vi "3DVisPrep.vi"() -> ()   [LabVIEW 2022 SP3]
uses:
  <vilib>/Utility/file.llb/Read From Spreadsheet File (DBL).vi
  <vilib>/Utility/file.llb/Write To Spreadsheet File (DBL).vi
panel:
  in  "reduce pts by factor of":u8=1
  out "Array":u8[][][](array[numeric])
  in  "Image Size":cluster{"Width":u32, "Height":u32}
  in  "name of saved file":string="test"
  out "Pict Images (if any)":picture[](array[picture])
  out "BMP Dimensions":T1(array[cluster])
  in  "Choose Directory of Files":path=path "C:/WINDOWS/DESKTOP/rri.eye"
  in  "How to save data":u16(ring) items=["X Y Z value + param in spreadsheet", "Save spreadsheet planes as 8 bit byte planes", "Save spreadsheet planes as single byte file", "save spreadsheet planes as 8 bit bitmaps", "Save RGB BMP planes as one 8 bit byte file (Ernie's BMP)", "Save RGB BMP planes as 8 bit BMP files (Ernie's BMP)", "Save RGB BMP planes as one 8 bit byte file specify pixels in X and Y (Fred's BMP)", "Convert eye file to 8 bit unsigned byte file. Reduce points if desired"]
  out "Dimensions (Z,Y,X)":i32[](array[numeric])
  in  "Number of files":i32
  in  "Root name of file":string="plane"
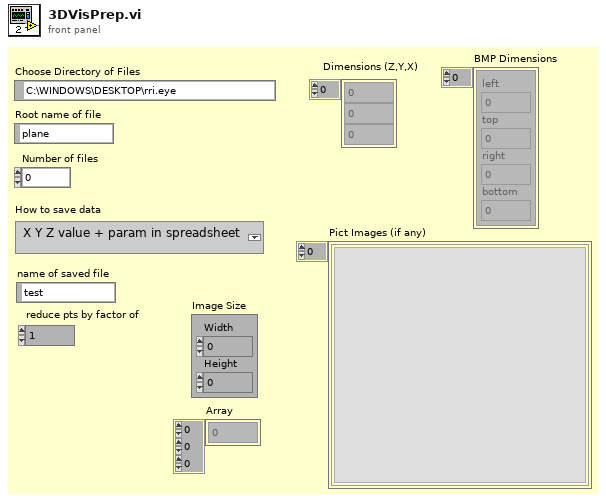
[diagram p1: front panel]
types:
  T1 = cluster{"left":i16, "top":i16, "right":i16, "bottom":i16}[]
  T2 = cluster{"left":i16, "top":i16, "right":i16, "bottom":i16}
  T3 = enum32{"existing file", "new file", "new or existing file", "existing dir", "new dir", "new or existing dir", "existing file (use LLBs)", "new file (use LLBs)", "new or existing file (use LLBs)", "new or existing file or directory (use LLBs)"}
  T4 = enum16{"open", "open or create", "create or replace", "create"}
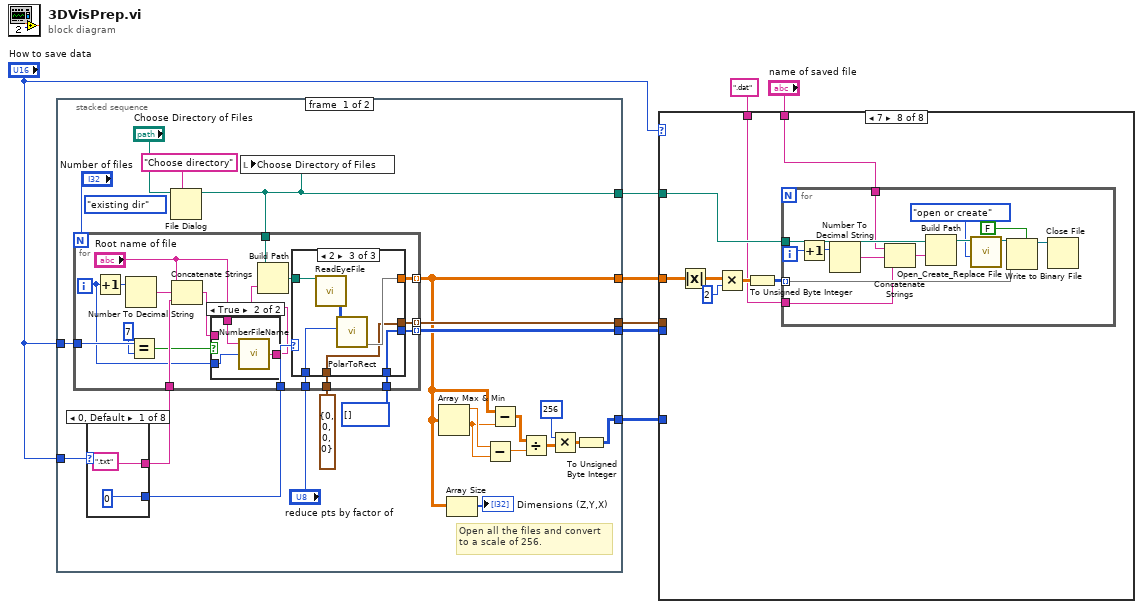
[diagram p0: block diagram]
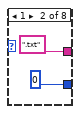
[diagram p2: hidden frame]
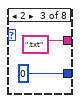
[diagram p3: hidden frame]
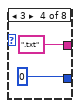
[diagram p4: hidden frame]
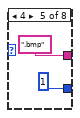
[diagram p5: hidden frame]
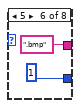
[diagram p6: hidden frame]
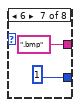
[diagram p7: hidden frame]
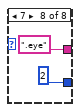
[diagram p8: hidden frame]
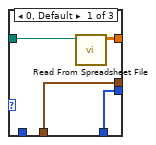
[diagram p10: hidden frame]
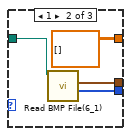
[diagram p11: hidden frame]
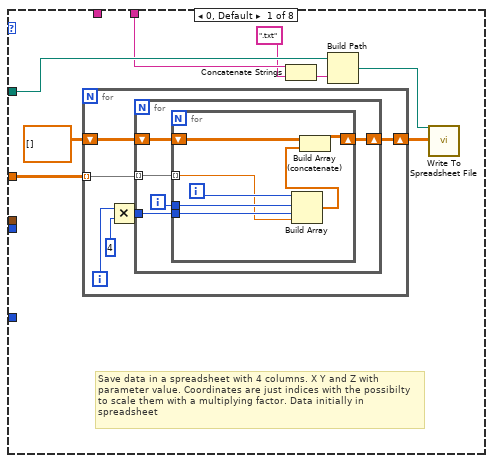
[diagram p13: hidden frame]
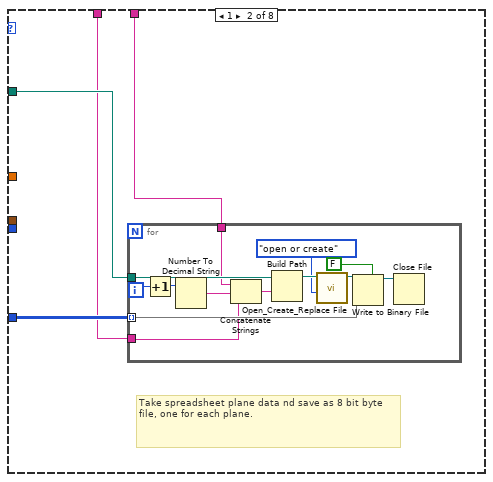
[diagram p14: hidden frame]
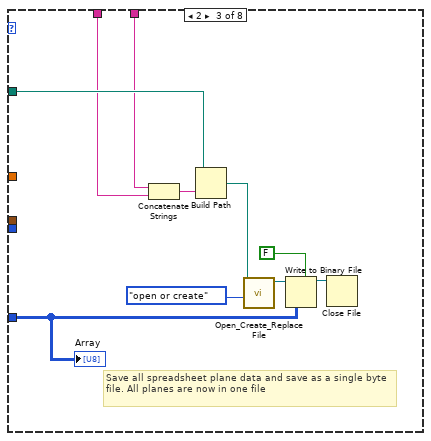
[diagram p15: hidden frame]
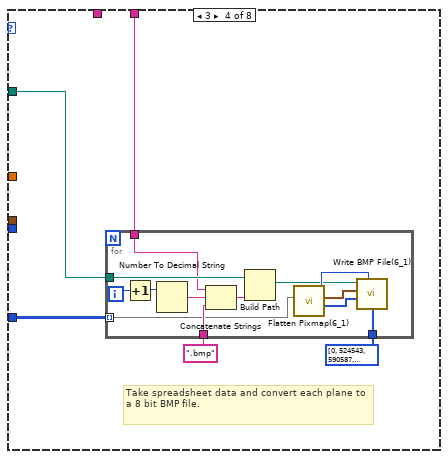
[diagram p16: hidden frame]
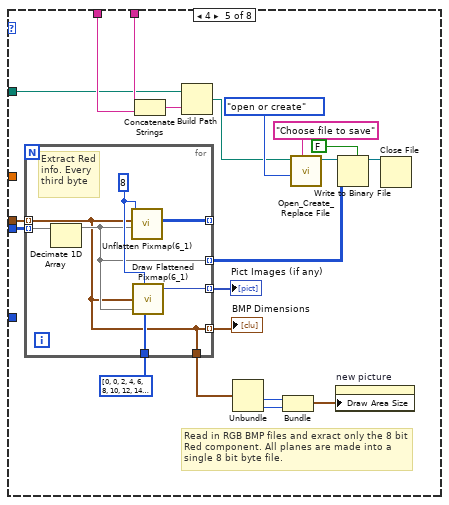
[diagram p17: hidden frame]
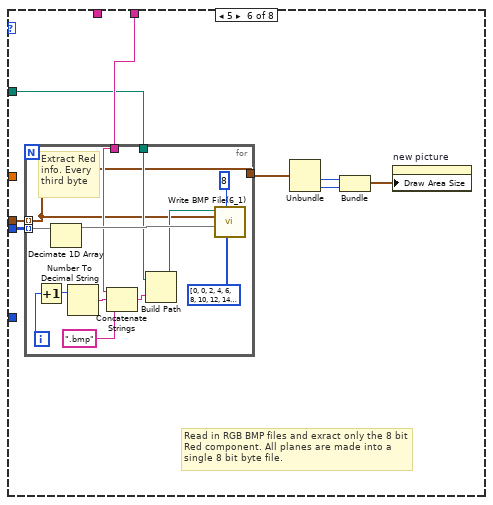
[diagram p18: hidden frame]
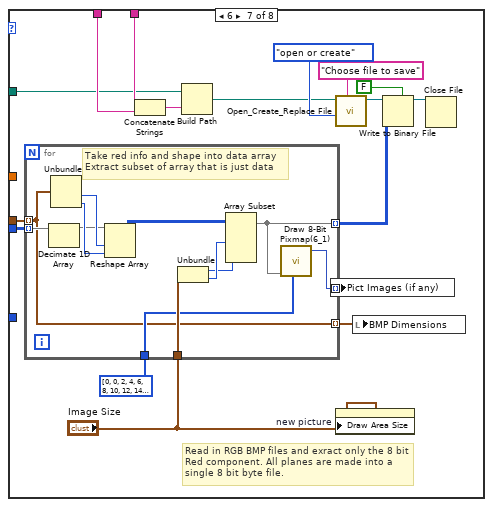
[diagram p19: hidden frame]
diagram:
  n1 = stacked-sequence {
    tunnel: [w27 _] -> w8
    tunnel: [w21 _] -> w7
    tunnel: [w17 _] -> w6
    tunnel: [w26 _] -> w5
    tunnel: [w25 _] -> w4
    tunnel: "How to save data" -> [w15 _]
    tunnel: "How to save data" -> [w10 _]
    frame #0 {
      (unwired) T3."existing dir" ("select mode (2)")
      # "Open all the files and convert\nto a scale of 256."
      n2 = case shown="0, Default" w15 {
        tunnel: [".txt" ".txt" ".txt" ".txt" ".bmp" ".bmp" ".bmp" ".eye"] -> w14
        tunnel: [0 0 0 0 1 1 1 2] -> w13
        frame 0, Default {
        }
        frame 1 {
        }
        frame 2 {
        }
        frame 3 {
        }
        frame 4 {
        }
        frame 5 {
        }
        frame 6 {
        }
        frame 7 {
        }
      }
      n3 = File Dialog(7:"Choose directory" ("prompt"), 11:"Choose Directory of Files") -> (3:w27:path)  [unwired: 5 in, 3 out]
      n4 = for {
        N: "Number of files" -> [_]
        tunnel: w27 -> [w65]
        tunnel: [w63] -> w21 mode=indexing
        tunnel: [w62] -> w26 mode=indexing
        tunnel: [w61] -> w25 mode=indexing
        tunnel: w14 -> [w60]
        tunnel: w13 -> [w59]
        tunnel: u8[] [] ("Array Constant") -> [w58]
        tunnel: T2 {"left"=0, "top"=0, "right"=0, "bottom"=0} ("rect") -> [w57]
        tunnel: w10 -> [w55]
        tunnel: "reduce pts by factor of" -> [w49]
        i -> [w50]
        n5 = Increment(x=w50) -> (x+1=w51:i32)
        n6 = Number To Decimal String(number=w51) -> (decimal integer string=w66:string)  [unwired: 1 in]
        n7 = Equal?(x=w55, y=7) -> (x = y?=w56:bool)
        n8 = Concatenate Strings("Root name of file", w66, w60) -> (w53:string)
        n9 = case shown="True" w56 {
          tunnel: [w67 w70] -> w48
          tunnel: w53 -> [w67 _]
          tunnel: "Root name of file" -> [_ w69]
          tunnel: w50 -> [_ w68]
          frame False {
          }
          frame True {
            n10 = call "NumberFileName.vi"("File number"=w68, "file name"=w69) -> ("Numbered File"=w70:string)  [unwired: 1 in]
          }
        }
        n11 = Build Path(base path=w65, name or relative path=w48) -> (appended path=w64:path)
        n12 = case shown="2" w59 {
          tunnel: w64 -> [w74 w78 w84]
          tunnel: [w73 dbl[][] [] ("Array Constant") w82] -> w63
          tunnel: [w72 w77 w81] -> w62
          tunnel: [w71 w75 w80] -> w61
          tunnel: w58 -> [w72 _ w81]
          tunnel: w57 -> [w71 _ w80]
          tunnel: w49 -> [_ _ w79]
          frame 0, Default {
            n13 = call-poly <vilib>:"Read From Spreadsheet File.vi"("file path (dialog if empty)"=w74) -> ("all rows"=w73:dbl[][])  [unwired: 6 in, 4 out]
          }
          frame 1 {
            n14 = call <vilib>:"Read BMP File(6_1).vi"("path to BMP file"=w78) -> ("flattened image data"=w77:u8[], "rect"=w75:T2)  [unwired: 5 in, 4 out]
          }
          frame 2 {
            n15 = call "ReadEyeFile.vi"("new file path"=w84) -> ("2-D data array"=w83:i16[][])  [unwired: 10 in, 8 out]
            n16 = call "PolarToRect.vi"("c m/s"=w79, "array dims"=w83) -> (0:w82)  [unwired: 3 in, 6 out]
          }
        }
      }
      n17 = local write "Choose Directory of Files"(w27) -> ()
      n18 = Array Max & Min(array=w21) -> (max value=w24:dbl, min value=w23:dbl)  [unwired: 2 out]
      n19 = Array Size(array=w21) -> (size(s)=→"Dimensions (Z,Y,X)":i32[])
      n20 = Subtract(x=w24, y=w23) -> (x-y=w22:dbl)
      n21 = Subtract(x=w21, y=w23) -> (x-y=w20:dbl[][][])
      n22 = Divide(x=w20, y=w22) -> (x/y=w19:dbl[][][])
      n23 = Multiply(x=256, y=w19) -> (x*y=w16:dbl[][][])
      n24 = To Unsigned Byte Integer(number=w16) -> (unsigned 8bit integer=w17:u8[][][])
    }
    frame #1 {
    }
  }
  n25 = case shown="7" "How to save data" {
    tunnel: w8 -> [w89 w114 w133 w142 w162 w183 w210 w235]
    tunnel: w7 -> [w90 _ _ _ _ _ _ w240]
    tunnel: w6 -> [_ w113 w129 w139 _ _ _ _]
    tunnel: w5 -> [_ _ _ _ w175 w190 w220 _]
    tunnel: w4 -> [_ _ _ _ w174 w189 w219 _]
    tunnel: "name of saved file" -> [w87 w112 w132 w138 w164 w184 w212 w234]
    tunnel: ".dat" -> [_ w111 w131 _ w163 _ w211 w233]
    frame 0, Default {
      # "Save data in a spreadsheet with 4 columns. X Y and Z with parameter value. Coordinates are just indices with the possibilty\nto scale them with a multiplying factor. Data initially in spreadsheet"
      n26 = for {
        shift-right: [w98] -> w91
        shift-left: dbl[][] [] ("Array Constant") -> [w97]
        tunnel: w90 -> [w93] mode=indexing
        i -> [w95]
        n27 = Multiply(x=w95, y=4) -> (x*y=w94:i32)
        n28 = for {
          tunnel: w93 -> [w103] mode=indexing
          tunnel: w94 -> [w101]
          shift-right: [w100] -> w98
          shift-left: w97 -> [w99]
          i -> [w102]
          n29 = for {
            tunnel: w103 -> [w107] mode=indexing
            tunnel: w102 -> [w109]
            tunnel: w101 -> [w110]
            shift-right: [w105] -> w100
            shift-left: w99 -> [w106]
            i -> [w108]
            n30 = Build Array(w108, w109, w110, w107) -> (w104:dbl[])
            n31 = Build Array (concatenate)(w106, w104) -> (w105:dbl[][])
          }
        }
      }
      n32 = Concatenate Strings(w87, ".txt") -> (w86:string)
      n33 = Build Path(base path=w89, name or relative path=w86) -> (appended path=w88:path)
      n34 = call-poly <vilib>:"Write To Spreadsheet File.vi"("2D data"=w91, "file path (dialog if empty)"=w88) -> ()  [unwired: 6 in, 1 out]
    }
    frame 1 {
      # "Take spreadsheet plane data nd save as 8 bit byte file, one for each plane."
      n35 = for {
        tunnel: w113 -> [w121] mode=indexing
        tunnel: w114 -> [w120]
        tunnel: w112 -> [w119]
        tunnel: w111 -> [w117]
        i -> [w127]
        n36 = Increment(x=w127) -> (x+1=w126:i32)
        n37 = Number To Decimal String(number=w126) -> (decimal integer string=w118:string)  [unwired: 1 in]
        n38 = Concatenate Strings(w119, w118, w117) -> (w116:string)
        n39 = Build Path(base path=w120, name or relative path=w116) -> (appended path=w125:path)
        n40 = call <vilib>:"Open_Create_Replace File.vi"("function (open:0)"=T4."open or create", "file path"=w125) -> ("refnum"=w124:refnum<file>)  [unwired: 6 in, 3 out]
        n41 = Write to Binary File(file (use dialog)=w124, data=w121, 5:FALSE ("prepend array or string size? (T)")) -> (refnum out=w123:refnum<file>)  [unwired: 3 in, 2 out]
        n42 = Close File(refnum=w123) -> ()  [unwired: 1 in, 2 out]
      }
    }
    frame 2 {
      # "Save all spreadsheet plane data and save as a single byte file. All planes are now in one file"
      n43 = Concatenate Strings(w132, w131) -> (w134:string)
      n44 = Build Path(base path=w133, name or relative path=w134) -> (appended path=w130:path)
      n45 = call <vilib>:"Open_Create_Replace File.vi"("function (open:0)"=T4."open or create", "file path"=w130) -> ("refnum"=w136:refnum<file>)  [unwired: 6 in, 3 out]
      n46 = Write to Binary File(file (use dialog)=w136, data=w129, 5:FALSE ("prepend array or string size? (T)")) -> (refnum out=w137:refnum<file>)  [unwired: 3 in, 2 out]
      n47 = Close File(refnum=w137) -> ()  [unwired: 1 in, 2 out]
      "Array" <- w129
    }
    frame 3 {
      # "Take spreadsheet data and convert each plane to a 8 bit BMP file."
      n48 = for {
        tunnel: w139 -> [w147] mode=indexing
        tunnel: w142 -> [w153]
        tunnel: ".bmp" -> [w151]
        tunnel: u32[] [0, 524543, 590587, 591095, 657139, 657647, 723691, 724455, 790500, 791008, 857052, 923096, 923604, 989648, 990156, 1056200, 1056708, 1122752, 1123516, 1189560, 1255604, 1256113, 1322157, 1322665, 1388709, 1389217, 1455261, 1521305, 1521816, 1588120, 1588631, 1654678, 1655190, 1721237, 1721748, 1787796, 1853843, 1854354, 1920402, 1920913, 1987216, 1987728, 2053775, 2054286, 2120334, 2186381, 2186892, 2252940, 2253451, 2319498, 2320009, 2386313, 2386824, 2452871, 2518919, 2519430, 2585477, 2585989, 2652036, 2652547, 2718595, 2719106, 2785409, 2851457, 2851968, 2918015, 2918527, 2984574, 2985085, 3051133, 3051644, 3117691, 3183739, 3184250, 3250553, 3251065, 3317112, 3317623, 3383671, 3449718, 3450229, 3516277, 3516788, 3582835, 3583347, 3649650, 3650161, 3716209, 3782256, 3782767, 3848815, 3849326, 3915373, 3915885, 3981932, 3982443, 4048746, 4114794, 4115305, 4181352, 4181864, 4247911, 4248422, 4314470, 4314981, 4381028, 4447076, 4447843, 4513890, 4514402, 4580449, 4580960, 4647008, 4647519, 4713566, 4779614, 4780125, 4846172, 4846940, 4912987, 4913498, 4979546, 5045593, 5046104, 5111128, 5110615, 5175638, 5175126, 5240149, 5239636, 5304660, 5369683, 5369170, 5434450, 5433937, 5498960, 5498448, 5563471, 5562958, 5627982, 5693005, 5823564, 5888587, 6019147, 6084170, 6214729, 6279753, 6410312, 6475335, 6605895, 6670918, 6801477, 6866757, 6997316, 7062339, 7192899, 7257922, 7388481, 7453505, 7584064, 7649087, 7779647, 7844670, 7909693, 8040253, 8105276, 8235835, 8300859, 8431418, 8496441, 8627257, 8692280, 8822839, 8887863, 9018422, 9083445, 9214005, 9279028, 9409587, 9474611, 9605170, 9670193, 9800753, 9865776, 9996335, 10061359, 10126382, 10256941, 10321964, 10452780, 10517803, 10648362, 10713386, 10843945, 10908968, 11039528, 11104551, 11235110, 11300134, 11430693, 11495716, 11626276, 11691299, 11821858, 11886882, 12017441, 12082464, 12213024, 12278303, 12343326, 12473886, 12538909, 12669468, 12734492, 12865051, 12930074, 13060634, 13125657, 13256216, 13321240, 13451799, 13516822, 13647382, 13712405, 13842964, 13907988, 14038803, 14103826, 14234386, 14299409, 14429968, 14494992, 14560015, 14690574, 14755597, 14886157, 14951180, 15081739, 15146763, 15277322, 15342345, 15472905, 15537928, 15668487, 15733511, 15864326, 15929349, 16059909, 16124932, 16255491, 16320515, 16451074, 16516097, 16646657, 16711680, 16711680] -> [w144]
        tunnel: w138 -> [w143]
        i -> [w155]
        n49 = Increment(x=w155) -> (x+1=w154:i32)
        n50 = Number To Decimal String(number=w154) -> (decimal integer string=w152:string)  [unwired: 1 in]
        n51 = Concatenate Strings(w143, w152, w151) -> (w150:string)
        n52 = Build Path(base path=w153, name or relative path=w150) -> (appended path=w148:path)
        n53 = call <vilib>:"Flatten Pixmap(6_1).vi"("8-bit pixmap"=w147) -> ("flattened image data"=w145:u8[], "bounds"=w146:T2, "bit depth"=w149:u8)  [unwired: 8 in]
        n54 = call <vilib>:"Write BMP File(6_1).vi"("color table"=w144, "depth"=w149, "flattened image data"=w145, "rect"=w146, "path to BMP file"=w148) -> ()  [unwired: 5 in, 2 out]
      }
    }
    frame 4 {
      # "Read in RGB BMP files and exract only the 8 bit Red component. All planes are made into a single 8 bit byte file."
      n55 = for {
        tunnel: w175 -> [w181] mode=indexing
        tunnel: w174 -> [w176] mode=indexing
        tunnel: [w180] -> w167 mode=indexing
        tunnel: [w176] -> w173 mode=indexing
        tunnel: u32[] [0, 0, 2, 4, 6, 8, 10, 12, 14, 16, 18, 20, 22, 24, 26, 28, 30, 32, 34, 36, 38, 40, 42, 44, 46, 48, 50, 52, 54, 56, 58, 60, 62, 64, 66, 68, 70, 72, 74, 76, 78, 80, 82, 84, 86, 88, 90, 92, 94, 96, 98, 100, 102, 104, 106, 108, 110, 112, 114, 116, 118, 120, 122, 124, 126, 128, 130, 132, 134, 136, 138, 140, 142, 144, 146, 148, 150, 152, 154, 156, 158, 160, 162, 164, 166, 168, 170, 172, 174, 176, 178, 180, 182, 184, 186, 188, 190, 192, 194, 196, 198, 200, 202, 204, 206, 208, 210, 212, 214, 216, 218, 220, 222, 224, 226, 228, 230, 232, 234, 236, 238, 240, 242, 244, 246, 248, 250, 252, 255, 131839, 263423, 395007, 526591, 658175, 789759, 921343, 1052927, 1184511, 1316095, 1447679, 1579263, 1710847, 1842431, 1974015, 2105599, 2237183, 2368767, 2500351, 2631935, 2763519, 2895103, 3026687, 3158271, 3289855, 3421439, 3553023, 3684607, 3816191, 3947775, 4079359, 4210943, 4342527, 4474111, 4605695, 4737279, 4868863, 5000447, 5132031, 5263615, 5395199, 5526783, 5658367, 5789951, 5921535, 6053119, 6184703, 6316287, 6447871, 6579455, 6711039, 6842623, 6974207, 7105791, 7237375, 7368959, 7500543, 7632127, 7763711, 7895295, 8026879, 8158463, 8290047, 8421631, 8553215, 8684799, 8816383, 8947967, 9079551, 9211135, 9342719, 9474303, 9605887, 9737471, 9869055, 10000639, 10132223, 10263807, 10395391, 10526975, 10658559, 10790143, 10921727, 11053311, 11184895, 11316479, 11448063, 11579647, 11711231, 11842815, 11974399, 12105983, 12237567, 12369151, 12500735, 12632319, 12763903, 12895487, 13027071, 13158655, 13290239, 13421823, 13553407, 13684991, 13816575, 13948159, 14079743, 14211327, 14342911, 14474495, 14606079, 14737663, 14869247, 15000831, 15132415, 15263999, 15395583, 15527167, 15658751, 15790335, 15921919, 16053503, 16185087, 16316671, 16448255, 16579839, 16711680] ("Array 3") -> [w179]
        tunnel: [w178] -> _ mode=indexing
        tunnel: [w177] -> w166 mode=indexing
        tunnel: [w176] -> w158
        w182 = 8
        # "Extract Red\ninfo. Every \nthird byte"
        n56 = Decimate 1D Array(w181) -> (w180:u8[])  [unwired: 2 out]
        n57 = call <vilib>:"Unflatten Pixmap(6_1).vi"("flattened image data"=w180, "rect"=w176, "depth"=w182) -> ("8-bit pixmap"=w178:u8[][])  [unwired: 4 in, 4 out]
        n58 = call <vilib>:"Draw Flattened Pixmap(6_1).vi"("bit depth(8)"=w182, "rect"=w176, "flattened pixmap data"=w180, "color table"=w179) -> ("new picture"=w177:picture)  [unwired: 5 in]
      }
      "Pict Images (if any)" <- w166
      "BMP Dimensions" <- w173
      n59 = Concatenate Strings(w164, w163) -> (w165:string)
      n60 = Build Path(base path=w162, name or relative path=w165) -> (appended path=w161:path)
      n61 = Unbundle(w158) -> ("right"=w160:i16, "bottom"=w159:i16)  [unwired: 2 out]
      n62 = Bundle("right"=w160, "bottom"=w159) -> (w157:cluster{"right":i16, "bottom":i16})  [unwired: 1 in]
      n63 = call <vilib>:"Open_Create_Replace File.vi"("prompt"="Choose file to save", "function (open:0)"=T4."open or create", "file path"=w161) -> ("refnum"=w171:refnum<file>)  [unwired: 5 in, 3 out]
      n64 = property on="new picture" class="Pict"("Draw Area Size"=w157) -> ()  [unwired: 2 in, 2 out]
      n65 = Write to Binary File(file (use dialog)=w171, data=w167, 5:FALSE ("prepend array or string size? (T)")) -> (refnum out=w170:refnum<file>)  [unwired: 3 in, 2 out]
      n66 = Close File(refnum=w170) -> ()  [unwired: 1 in, 2 out]
    }
    frame 5 {
      # "Read in RGB BMP files and exract only the 8 bit Red component. All planes are made into a single 8 bit byte file."
      n67 = for {
        tunnel: w190 -> [w203] mode=indexing
        tunnel: w189 -> [w191] mode=indexing
        tunnel: [w191] -> w186
        tunnel: w184 -> [w194]
        tunnel: w183 -> [w193]
        i -> [w196]
        # "Extract Red\ninfo. Every \nthird byte"
        n68 = Increment(x=w196) -> (x+1=w198:i32)
        n69 = Decimate 1D Array(w203) -> (w202:u8[])  [unwired: 2 out]
        n70 = Number To Decimal String(number=w198) -> (decimal integer string=w199:string)  [unwired: 1 in]
        n71 = Concatenate Strings(w194, w199, ".bmp") -> (w200:string)
        n72 = Build Path(base path=w193, name or relative path=w200) -> (appended path=w192:path)
        n73 = call <vilib>:"Write BMP File(6_1).vi"("color table"=u32[] [0, 0, 2, 4, 6, 8, 10, 12, 14, 16, 18, 20, 22, 24, 26, 28, 30, 32, 34, 36, 38, 40, 42, 44, 46, 48, 50, 52, 54, 56, 58, 60, 62, 64, 66, 68, 70, 72, 74, 76, 78, 80, 82, 84, 86, 88, 90, 92, 94, 96, 98, 100, 102, 104, 106, 108, 110, 112, 114, 116, 118, 120, 122, 124, 126, 128, 130, 132, 134, 136, 138, 140, 142, 144, 146, 148, 150, 152, 154, 156, 158, 160, 162, 164, 166, 168, 170, 172, 174, 176, 178, 180, 182, 184, 186, 188, 190, 192, 194, 196, 198, 200, 202, 204, 206, 208, 210, 212, 214, 216, 218, 220, 222, 224, 226, 228, 230, 232, 234, 236, 238, 240, 242, 244, 246, 248, 250, 252, 255, 131839, 263423, 395007, 526591, 658175, 789759, 921343, 1052927, 1184511, 1316095, 1447679, 1579263, 1710847, 1842431, 1974015, 2105599, 2237183, 2368767, 2500351, 2631935, 2763519, 2895103, 3026687, 3158271, 3289855, 3421439, 3553023, 3684607, 3816191, 3947775, 4079359, 4210943, 4342527, 4474111, 4605695, 4737279, 4868863, 5000447, 5132031, 5263615, 5395199, 5526783, 5658367, 5789951, 5921535, 6053119, 6184703, 6316287, 6447871, 6579455, 6711039, 6842623, 6974207, 7105791, 7237375, 7368959, 7500543, 7632127, 7763711, 7895295, 8026879, 8158463, 8290047, 8421631, 8553215, 8684799, 8816383, 8947967, 9079551, 9211135, 9342719, 9474303, 9605887, 9737471, 9869055, 10000639, 10132223, 10263807, 10395391, 10526975, 10658559, 10790143, 10921727, 11053311, 11184895, 11316479, 11448063, 11579647, 11711231, 11842815, 11974399, 12105983, 12237567, 12369151, 12500735, 12632319, 12763903, 12895487, 13027071, 13158655, 13290239, 13421823, 13553407, 13684991, 13816575, 13948159, 14079743, 14211327, 14342911, 14474495, 14606079, 14737663, 14869247, 15000831, 15132415, 15263999, 15395583, 15527167, 15658751, 15790335, 15921919, 16053503, 16185087, 16316671, 16448255, 16579839, 16711680] ("Array 3"), "depth"=u8 8, "flattened image data"=w202, "rect"=w191, "path to BMP file"=w192) -> ()  [unwired: 5 in, 2 out]
      }
      n74 = Unbundle(w186) -> ("right"=w188:i16, "bottom"=w187:i16)  [unwired: 2 out]
      n75 = Bundle("right"=w188, "bottom"=w187) -> (w185:cluster{"right":i16, "bottom":i16})  [unwired: 1 in]
      n76 = property on="new picture" class="Pict"("Draw Area Size"=w185) -> ()  [unwired: 2 in, 2 out]
    }
    frame 6 {
      # "Read in RGB BMP files and exract only the 8 bit Red component. All planes are made into a single 8 bit byte file."
      n77 = for {
        tunnel: w220 -> [w227] mode=indexing
        tunnel: w219 -> [w222] mode=indexing
        tunnel: u32[] [0, 0, 2, 4, 6, 8, 10, 12, 14, 16, 18, 20, 22, 24, 26, 28, 30, 32, 34, 36, 38, 40, 42, 44, 46, 48, 50, 52, 54, 56, 58, 60, 62, 64, 66, 68, 70, 72, 74, 76, 78, 80, 82, 84, 86, 88, 90, 92, 94, 96, 98, 100, 102, 104, 106, 108, 110, 112, 114, 116, 118, 120, 122, 124, 126, 128, 130, 132, 134, 136, 138, 140, 142, 144, 146, 148, 150, 152, 154, 156, 158, 160, 162, 164, 166, 168, 170, 172, 174, 176, 178, 180, 182, 184, 186, 188, 190, 192, 194, 196, 198, 200, 202, 204, 206, 208, 210, 212, 214, 216, 218, 220, 222, 224, 226, 228, 230, 232, 234, 236, 238, 240, 242, 244, 246, 248, 250, 252, 255, 131839, 263423, 395007, 526591, 658175, 789759, 921343, 1052927, 1184511, 1316095, 1447679, 1579263, 1710847, 1842431, 1974015, 2105599, 2237183, 2368767, 2500351, 2631935, 2763519, 2895103, 3026687, 3158271, 3289855, 3421439, 3553023, 3684607, 3816191, 3947775, 4079359, 4210943, 4342527, 4474111, 4605695, 4737279, 4868863, 5000447, 5132031, 5263615, 5395199, 5526783, 5658367, 5789951, 5921535, 6053119, 6184703, 6316287, 6447871, 6579455, 6711039, 6842623, 6974207, 7105791, 7237375, 7368959, 7500543, 7632127, 7763711, 7895295, 8026879, 8158463, 8290047, 8421631, 8553215, 8684799, 8816383, 8947967, 9079551, 9211135, 9342719, 9474303, 9605887, 9737471, 9869055, 10000639, 10132223, 10263807, 10395391, 10526975, 10658559, 10790143, 10921727, 11053311, 11184895, 11316479, 11448063, 11579647, 11711231, 11842815, 11974399, 12105983, 12237567, 12369151, 12500735, 12632319, 12763903, 12895487, 13027071, 13158655, 13290239, 13421823, 13553407, 13684991, 13816575, 13948159, 14079743, 14211327, 14342911, 14474495, 14606079, 14737663, 14869247, 15000831, 15132415, 15263999, 15395583, 15527167, 15658751, 15790335, 15921919, 16053503, 16185087, 16316671, 16448255, 16579839, 16711680] ("Array 3") -> [w224]
        tunnel: [w223] -> w208 mode=indexing
        tunnel: [w225] -> w207 mode=indexing
        tunnel: "Image Size" -> [w232]
        tunnel: [w222] -> w205 mode=indexing
        # "Take red info and shape into data array\nExtract subset of array that is just data"
        n78 = Decimate 1D Array(w227) -> (w226:u8[])  [unwired: 2 out]
        n79 = Unbundle(w222) -> ("right"=w231:i16, "bottom"=w230:i16)  [unwired: 2 out]
        n80 = Reshape Array(w226, w231, w230) -> (w229:u8[][])
        n81 = Unbundle(w232) -> ("Width"=w221:u32, "Height"=w228:u32)
        n82 = Array Subset(array=w229, length (row)=w228, length (col)=w221) -> (w225:u8[][])  [unwired: 2 in]
        n83 = call <vilib>:"Draw 8-Bit Pixmap(6_1).vi"("data"=w225, "color table"=w224) -> ("new picture"=w223:picture)  [unwired: 7 in]
      }
      n84 = Concatenate Strings(w212, w211) -> (w213:string)
      n85 = Build Path(base path=w210, name or relative path=w213) -> (appended path=w209:path)
      n86 = local write "Pict Images (if any)"(w208) -> ()
      n87 = call <vilib>:"Open_Create_Replace File.vi"("prompt"="Choose file to save", "function (open:0)"=T4."open or create", "file path"=w209) -> ("refnum"=w217:refnum<file>)  [unwired: 5 in, 3 out]
      n88 = property on="new picture" class="Pict"("Draw Area Size"="Image Size") -> ()  [unwired: 2 in, 2 out]
      n89 = local write "BMP Dimensions"(w205) -> ()
      n90 = Write to Binary File(file (use dialog)=w217, data=w207, 5:FALSE ("prepend array or string size? (T)")) -> (refnum out=w216:refnum<file>)  [unwired: 3 in, 2 out]
      n91 = Close File(refnum=w216) -> ()  [unwired: 1 in, 2 out]
    }
    frame 7 {
      n92 = Absolute Value(x=w240) -> (abs(x)=w238:dbl[][][])
      n93 = Multiply(x=w238, y=2) -> (x*y=w237:dbl[][][])
      n94 = To Unsigned Byte Integer(number=w237) -> (unsigned 8bit integer=w236:u8[][][])
      n95 = for {
        tunnel: w236 -> [w247] mode=indexing
        tunnel: w235 -> [w246]
        tunnel: w234 -> [w245]
        tunnel: w233 -> [w243]
        i -> [w253]
        n96 = Increment(x=w253) -> (x+1=w252:i32)
        n97 = Number To Decimal String(number=w252) -> (decimal integer string=w244:string)  [unwired: 1 in]
        n98 = Concatenate Strings(w245, w244, w243) -> (w242:string)
        n99 = Build Path(base path=w246, name or relative path=w242) -> (appended path=w251:path)
        n100 = call <vilib>:"Open_Create_Replace File.vi"("function (open:0)"=T4."open or create", "file path"=w251) -> ("refnum"=w250:refnum<file>)  [unwired: 6 in, 3 out]
        n101 = Write to Binary File(file (use dialog)=w250, data=w247, 5:FALSE ("prepend array or string size? (T)")) -> (refnum out=w249:refnum<file>)  [unwired: 3 in, 2 out]
        n102 = Close File(refnum=w249) -> ()  [unwired: 1 in, 2 out]
      }
    }
  }
